vi "Query Numeric.vi"   [LabVIEW 2021, in "Yokogawa WT1800 Series.lvlib"]
doc: "Queries the specified numeric data output item."
uses:
  <instrlib>/Yokogawa WT1800 Series/Yokogawa WT1800 Series.lvlib
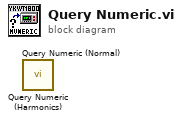
[diagram p0: block diagram]
diagram:
  n1 = call <instrlib>:"Query Numeric (Harmonics).vi"() -> ()  [unwired: 9 in, 3 out]
  n2 = call <instrlib>:"Query Numeric (Normal).vi"() -> ()  [unwired: 9 in, 3 out]
